vi "Vis To Table.vi"(7 "Image Folder Path":path, 11 "Vis":refnum<class "Vi.lvclass">[](array[class])) -> (3 "Table":refnum<class "Bloc.lvclass">[](array[class]))   [LabVIEW 2021, in "TAF Proj Document Type.lvlib" / "Vi.lvclass"]
uses:
  <vilib>/Wovalab/AntiDoc/Document Type/Add-ons/LabVIEW TAF Project/Vi/Vi.lvclass
  C:/Program Files (x86)/National Instruments/LabVIEW 2021/vi.lib/Wovalab/AntiDoc/Bloc/Bloc.lvclass
  <vilib>/Wovalab/AsciiDoc for LabVIEW/Adoc-Bloc/Bloc.lvclass
  <vilib>/Wovalab/AsciiDoc for LabVIEW/Table/Table Attributes--cluster.ctl
  <vilib>/Wovalab/AsciiDoc for LabVIEW/Table/Frame--enum.ctl
  <vilib>/Wovalab/AsciiDoc for LabVIEW/Table/Grid--enum.ctl
  <vilib>/Wovalab/AsciiDoc for LabVIEW/Table/Stripes--enum.ctl
  <vilib>/Wovalab/AsciiDoc for LabVIEW/Table/Column Attributes--cluster.ctl
  <vilib>/Wovalab/AsciiDoc for LabVIEW/Table/Horizontal Alignment--enum.ctl
  <vilib>/Wovalab/AsciiDoc for LabVIEW/Table/Vertical Alignment--enum.ctl
  <vilib>/Wovalab/AsciiDoc for LabVIEW/Table/Style--enum.ctl
  <vilib>/Wovalab/AntiDoc/Bloc/Bloc.lvclass/Bloc.ctl
  <vilib>/Wovalab/AntiDoc/Document Type/Add-ons/LabVIEW TAF Project/Vi/Vi.lvclass/Vi.ctl
  <vilib>/Wovalab/AsciiDoc for LabVIEW/Table/Table.lvclass/Table.ctl
  <vilib>/Wovalab/AntiDoc/Bloc/Read Name.vi
  <vilib>/Wovalab/AsciiDoc for LabVIEW/Paragraph/Paragraph.lvclass
  C:/Program Files (x86)/National Instruments/LabVIEW 2021/vi.lib/Wovalab/AsciiDoc for LabVIEW/Adoc-Bloc/Bloc.lvclass
  <vilib>/Wovalab/AsciiDoc for LabVIEW/Table/Table.lvclass
  <vilib>/Wovalab/Asciidoc for LabVIEW/Image/Image.lvclass
  <vilib>/Wovalab/AntiDoc/Utilities/Utilities.lvlib
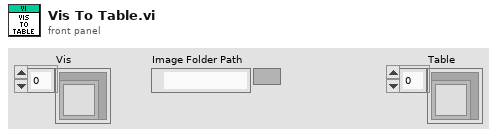
[diagram p1: front panel]
types:
  T1 = typedef "Wovalab_lib_AsciiDoctor.lvlib/Table.lvclass/Column Attributes--cluster.ctl" = cluster{"Width":u16, "Horizontal Alignment":T2, "Vertical Alignment":T3, "Style":T4}
  T2 = typedef "Wovalab_lib_AsciiDoctor.lvlib/Table.lvclass/Horizontal Alignment--enum.ctl" = enum16{"Left", "Center", "Right"}
  T3 = typedef "Wovalab_lib_AsciiDoctor.lvlib/Table.lvclass/Vertical Alignment--enum.ctl" = enum16{"Top", "Middle", "Bottom"}
  T4 = typedef "Wovalab_lib_AsciiDoctor.lvlib/Table.lvclass/Style--enum.ctl" = enum16{"None", "AsciiDoc", "Emphasis", "Header", "Literal", "Monospaced", "Strong", "Verse"}
  T5 = typedef "Wovalab_lib_AsciiDoctor.lvlib/Table.lvclass/Table Attributes--cluster.ctl" = cluster{"autowidth":bool, "Witdth":u8, "Frame":T6, "Grid":T7, "Stripes":T8}
  T6 = typedef "Wovalab_lib_AsciiDoctor.lvlib/Table.lvclass/Frame--enum.ctl" = enum16{"all", "topbot", "sides", "none"}
  T7 = typedef "Wovalab_lib_AsciiDoctor.lvlib/Table.lvclass/Grid--enum.ctl" = enum16{"all", "rows", "cols", "none"}
  T8 = typedef "Wovalab_lib_AsciiDoctor.lvlib/Table.lvclass/Stripes--enum.ctl" = enum16{"none", "even", "odd", "all", "hover"}
  T9 = typedef "imagedata.ctl" = cluster{"image type":i32, "image depth":i32, "image":u8[], "mask":u8[], "colors":u32[], "Rectangle":cluster{"left":i16, "top":i16, "right":i16, "bottom":i16}}
  T10 = enum16{"Share clones between instances", "Preallocate clone for each instance"}
  T11 = enum32{"invalid scope", "public", "private", "protected", "community"}
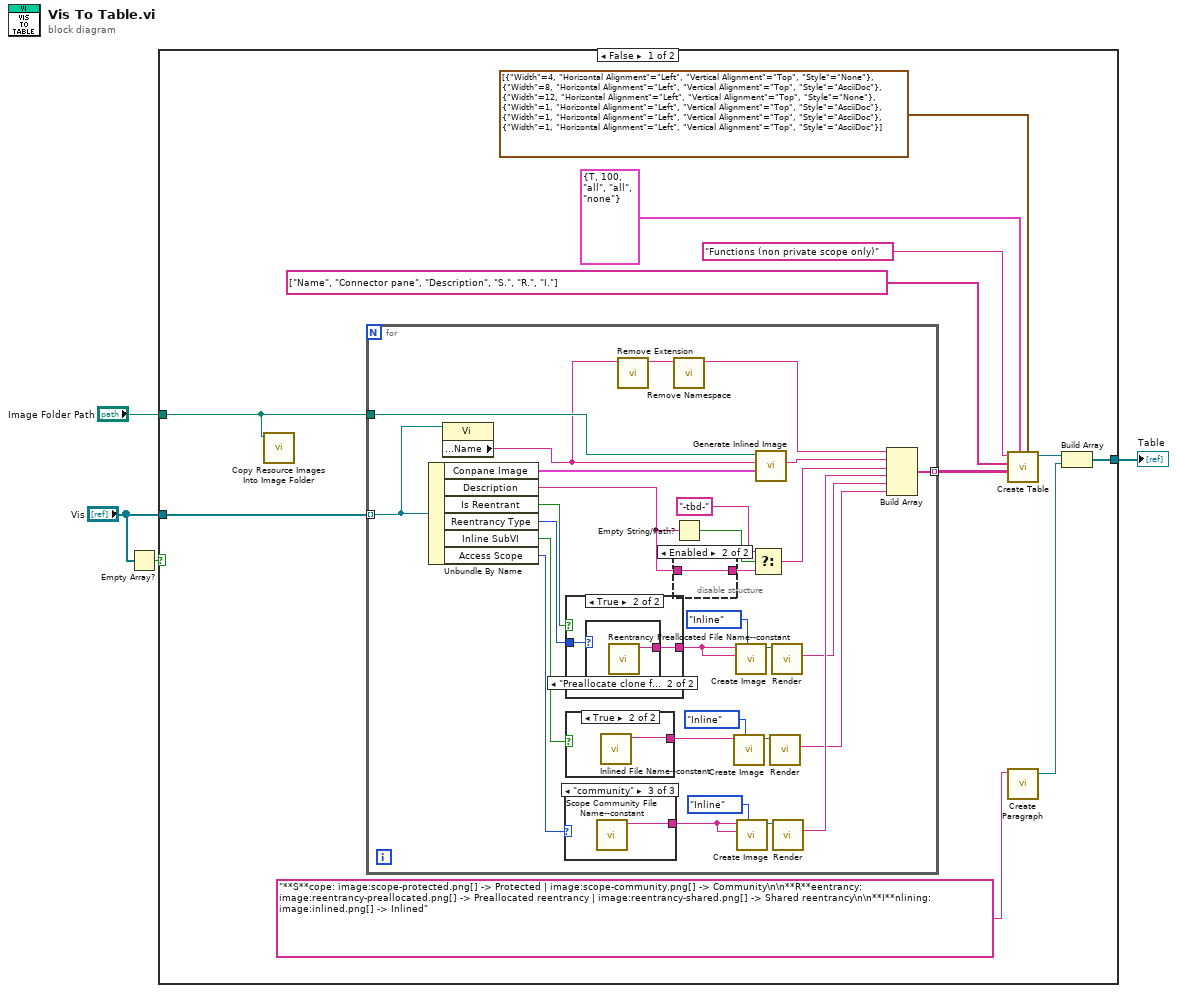
[diagram p0: block diagram]
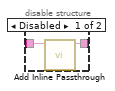
[diagram p2: hidden frame]
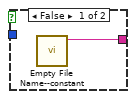
[diagram p3: hidden frame]
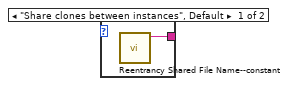
[diagram p4: hidden frame]
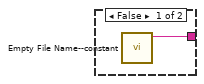
[diagram p5: hidden frame]
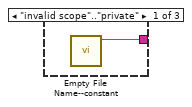
[diagram p6: hidden frame]
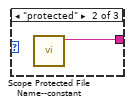
[diagram p7: hidden frame]
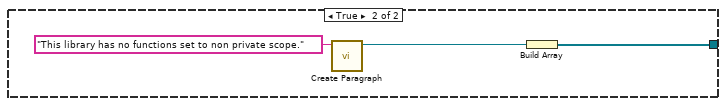
[diagram p8: hidden frame]
diagram:
  n1 = Empty Array?(array="Vis") -> (empty?=w1:bool)
  n2 = case shown="False" w1 {
    tunnel: "Vis" -> [w15 _]
    tunnel: "Image Folder Path" -> [w5 _]
    tunnel: [w6 w59] -> w3
    frame False {
      n3 = call <vilib>:"Copy Resource Images Into Image Folder.vi"("Image Folder Path"=w5) -> ()  [unwired: 9 in, 2 out]
      n4 = for {
        tunnel: w15 -> [w22] mode=indexing
        tunnel: w5 -> [w39]
        tunnel: [w44] -> w12 mode=indexing
        n5 = Unbundle By Name(w22) -> ("Conpane Image"=w38:T9, "Description"=w18:string, "Is Reentrant"=w41:bool, "Reentrancy Type"=w40:T10, "Inline SubVI"=w42:bool, "Access Scope"=w43:T11)
        n6 = property class="Vi"(reference=w22) -> ("Accessors:Name"=w20:string)  [unwired: 1 in, 2 out]
        n7 = case shown="\"community\"" w43 {
          tunnel: [w55 w56 w57] -> w34
          frame "invalid scope".."private" {
            n8 = call <vilib>:"Empty File Name--constant.vi"() -> ("Image File Name"=w55:string)  [unwired: 11 in]
          }
          frame "protected" {
            n9 = call <vilib>:"Scope Protected File Name--constant.vi"() -> ("Image File Name"=w56:string)  [unwired: 11 in]
          }
          frame "community" {
            n10 = call <vilib>:"Scope Community File Name--constant.vi"() -> ("Image File Name"=w57:string)  [unwired: 11 in]
          }
        }
        n11 = case shown="True" w41 {
          tunnel: [w48 w49] -> w28
          tunnel: w40 -> [_ w50]
          frame False {
            n12 = call <vilib>:"Empty File Name--constant.vi"() -> ("Image File Name"=w48:string)  [unwired: 11 in]
          }
          frame True {
            n13 = case shown="\"Preallocate clone for each instance\"" w50 {
              tunnel: [w51 w52] -> w49
              frame "Share clones between instances", Default {
                n14 = call <vilib>:"Reentrancy Shared File Name--constant.vi"() -> ("Image File Name"=w51:string)  [unwired: 11 in]
              }
              frame "Preallocate clone for each instance" {
                n15 = call <vilib>:"Reentrancy Preallocated File Name--constant.vi"() -> ("Image File Name"=w52:string)  [unwired: 11 in]
              }
            }
          }
        }
        n16 = case shown="True" w42 {
          tunnel: [w53 w54] -> w31
          frame False {
            n17 = call <vilib>:"Empty File Name--constant.vi"() -> ("Image File Name"=w53:string)  [unwired: 11 in]
          }
          frame True {
            n18 = call <vilib>:"Inlined File Name--constant.vi"() -> ("Image File Name"=w54:string)  [unwired: 11 in]
          }
        }
        n19 = call <vilib>:"Remove Extension.vi"("File Name"=w20) -> ("File Name Without Extension"=w21:string)  [unwired: 10 in]
        n20 = call <vilib>:"Remove Namespace.vi"("Vi Name"=w21) -> ("Vi Name Without Namespace"=w19:string)  [unwired: 10 in]
        n21 = Empty String/Path?(string/path=w18) -> (empty?=w27:bool)
        n22 = disable-structure shown="Enabled" {
          disable-tunnel: w18 -> [w46 w47]
          disable-tunnel: [w45 w47] -> w17
          frame Disabled {
            n23 = call <vilib>:"Add Inline Passthrough.vi"("String in"=w46) -> ("String out"=w45:string)  [unwired: 10 in]
          }
          frame Enabled {
          }
        }
        n24 = call <vilib>:"Create Image.vi"("Type"=enum16{"Block", "Inline"}."Inline", "Alt Text"=w31, "Image Path"=w31) -> ("Image out"=w32:refnum<class "Image.lvclass">)  [unwired: 7 in, 1 out]
        n25 = call <vilib>:"Create Image.vi"("Type"=enum16{"Block", "Inline"}."Inline", "Alt Text"=w28, "Image Path"=w28) -> ("Image out"=w30:refnum<class "Image.lvclass">)  [unwired: 7 in, 1 out]
        n26 = call <vilib>:"Create Image.vi"("Type"=enum16{"Block", "Inline"}."Inline", "Alt Text"=w34, "Image Path"=w34) -> ("Image out"=w36:refnum<class "Image.lvclass">)  [unwired: 7 in, 1 out]
        n27 = Select(t="-tbd-" ("Description Source"), s=w27, f=w17) -> (s? t:f=w26:string)
        n28 = call <vilib>:"Generate Inlined Image.vi"("empty"=w38, "Name"=w20, "Image Folder Path"=w39) -> ("Image String"=w37:string)  [unwired: 6 in, 2 out]
        n29 = call-dynamic "Render.vi"("Adoc-Image in"=w32) -> ("Output"=w23:string)  [unwired: 8 in, 2 out]
        n30 = call-dynamic "Render.vi"("Adoc-Image in"=w30) -> ("Output"=w24:string)  [unwired: 8 in, 2 out]
        n31 = call-dynamic "Render.vi"("Adoc-Image in"=w36) -> ("Output"=w25:string)  [unwired: 8 in, 2 out]
        n32 = Build Array(w19, w37, w26, w25, w24, w23) -> (w44:string[])
      }
      n33 = call <vilib>:"Create Table.vi"("Column Attributes"=T1[] [{"Width"=4, "Horizontal Alignment"=enum."Left", "Vertical Alignment"=enum."Top", "Style"=enum."None"}, {"Width"=8, "Horizontal Alignment"=enum."Left", "Vertical Alignment"=enum."Top", "Style"=enum."AsciiDoc"}, {"Width"=12, "Horizontal Alignment"=enum."Left", "Vertical Alignment"=enum."Top", "Style"=enum."None"}, {"Width"=1, "Horizontal Alignment"=enum."Left", "Vertical Alignment"=enum."Top", "Style"=enum."AsciiDoc"}, {"Width"=1, "Horizontal Alignment"=enum."Left", "Vertical Alignment"=enum."Top", "Style"=enum."AsciiDoc"}, {"Width"=1, "Horizontal Alignment"=enum."Left", "Vertical Alignment"=enum."Top", "Style"=enum."AsciiDoc"}], "Table Attributes"=T5 {"autowidth"=TRUE, "Witdth"=100, "Frame"=enum."all", "Grid"=enum."all", "Stripes"=enum."none"}, "Content"=w12, "Header"=string[] ["Name", "Connector pane", "Description", "S.", "R.", "I."], "Title"="Functions (non private scope only)") -> ("Table out"=w9:refnum<class "Table.lvclass">)  [unwired: 5 in, 1 out]
      n34 = call <vilib>:"Create Paragraph.vi"("Content"="**S**cope: image:scope-protected.png[] -> Protected | image:scope-community.png[] -> Community\n\n**R**eentrancy: image:reentrancy-preallocated.png[] -> Preallocated reentrancy | image:reentrancy-shared.png[] -> Shared reentrancy\n\n**I**nlining: image:inlined.png[] -> Inlined") -> ("Paragraph out"=w7:refnum<class "Paragraph.lvclass">)  [unwired: 9 in, 1 out]
      n35 = Build Array(w9, w7) -> (w6:refnum<class "Bloc.lvclass">[])
    }
    frame True {
      n36 = call <vilib>:"Create Paragraph.vi"("Content"="This library has no functions set to non private scope.") -> ("Paragraph out"=w60:refnum<class "Paragraph.lvclass">)  [unwired: 9 in, 1 out]
      n37 = Build Array(w60) -> (w59:refnum<class "Paragraph.lvclass">[])
    }
  }
  "Table" <- w3
